vi "SampleCalibrationImages.vi"(7 "TLCamera reference in":refnum<k24>, 8 "Error In":errorcluster, 10 "ExposureTime_us":u32, 11 "MotorController in":refnum<class "MotorController.lvclass">) -> (0 "Error Out":errorcluster, 3 "MotorController out":refnum<class "MotorController.lvclass">, 5 "TLCamera reference out":refnum<k24>)   [LabVIEW 2019]
uses:
  SampleCalibrationCalculationResults_cluster_typedef.ctl
  MotorController.lvclass
  C:/Users/jleeman/git_repos/CAxis_Machine/C-Axis LabView Controller/Library_X64/Thorlabs.TSI.TLCameraInterfaces.dll
  Library_X64/Thorlabs.TSI.TLCameraInterfaces.dll
  SampleCalibration_enum_states_typedef.ctl
  Axes_enum_typedef.ctl
panel:
  out "Calculation Results":T1
  in  "Calculate":bool
  in  "Go":bool
  in  "Jog Sample Steps":i16
  in  "Image":bool
  in  "Next":bool
  out "Image 2":T2(plugin-control)
  out "Image 1":T2(plugin-control)
  # "Sample Calibration"
  # "Take photos of the grid at 0 and 180 degree stage positions, then compare the offsets of the grid dots. Jog the stage and repeat as desired until sample holder is level with respect to the camera."
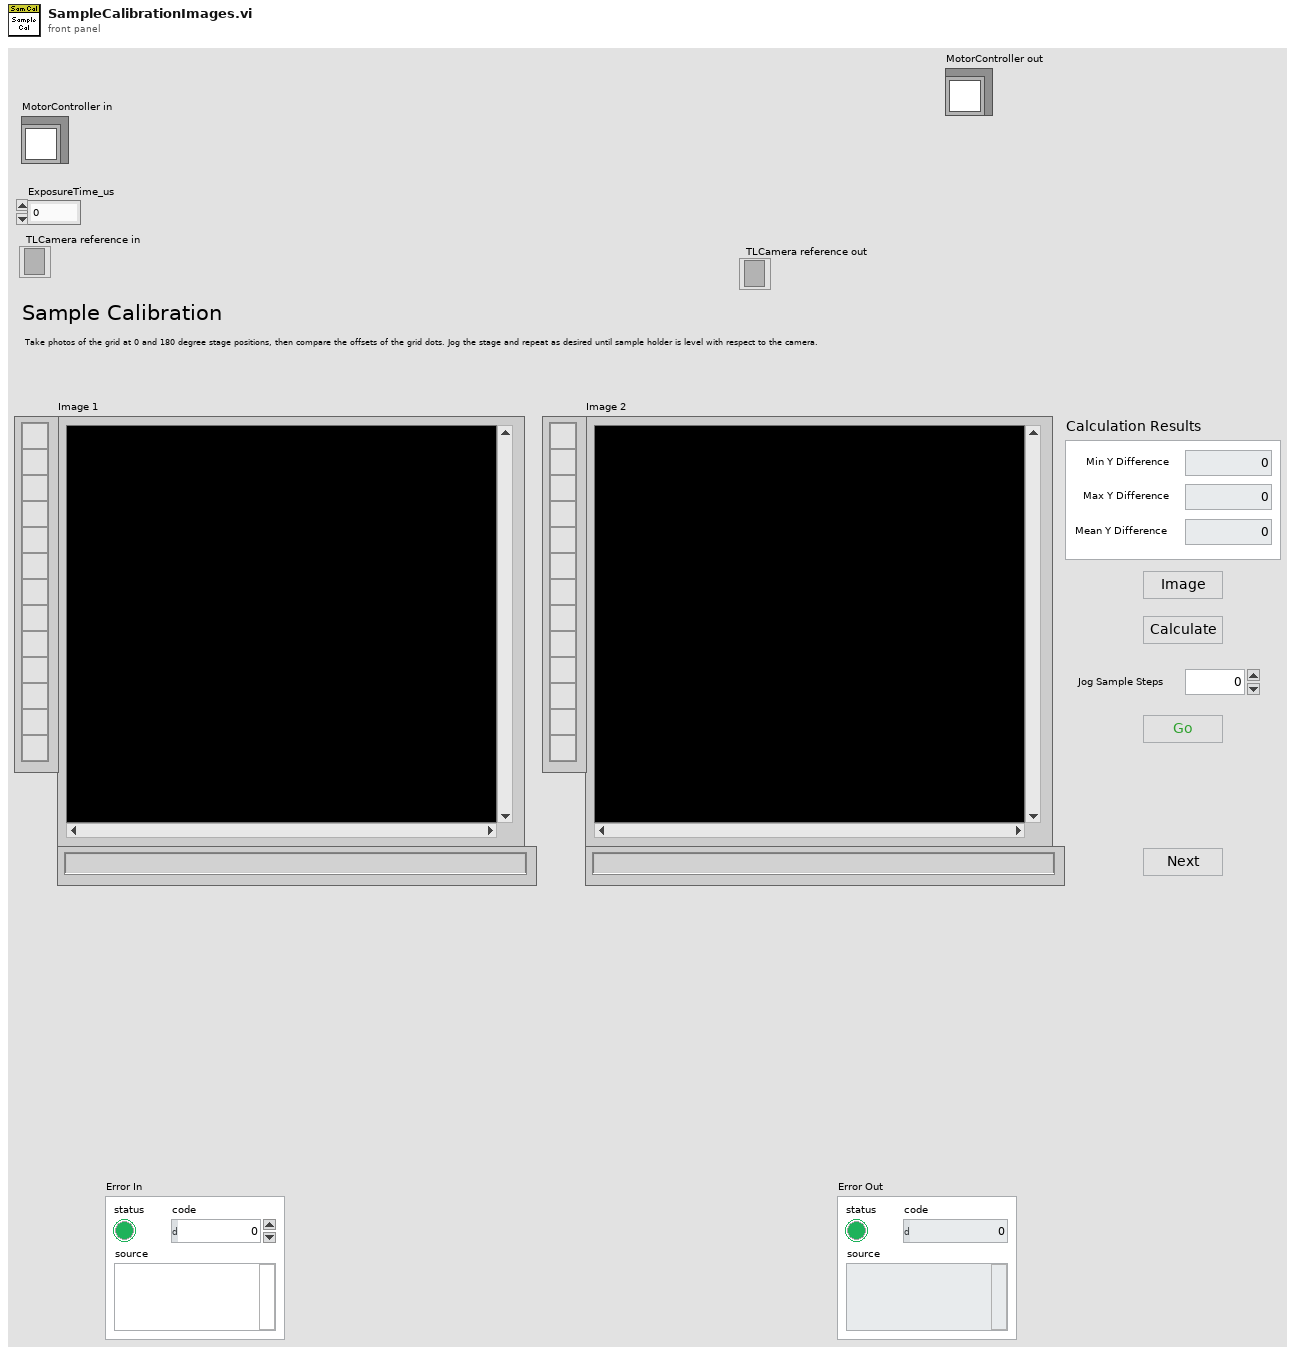
[diagram p1: front panel]
types:
  T1 = typedef "SampleCalibrationCalculationResults_cluster_typedef.ctl" = cluster{"Mean Y Difference":dbl, "Max Y Difference":dbl, "Min Y Difference":dbl}
  T2 = typedef "IMAQ Image.ctl" = refnum<image>
  T3 = typedef "Image Type" = u32
  T4 = enum8{"Enabled", "Disabled", "Disabled and Grayed Out"}
  T5 = typedef "SampleCalibration_enum_states_typedef.ctl" = enum16{"Initialize", "Move", "Capture", "Calculate", "Wait", "Shutdown"}
  T6 = typedef "Axes_enum_typedef.ctl" = enum16{"Polarizer 1", "Polarizer 2", "Sample", "Stage"}
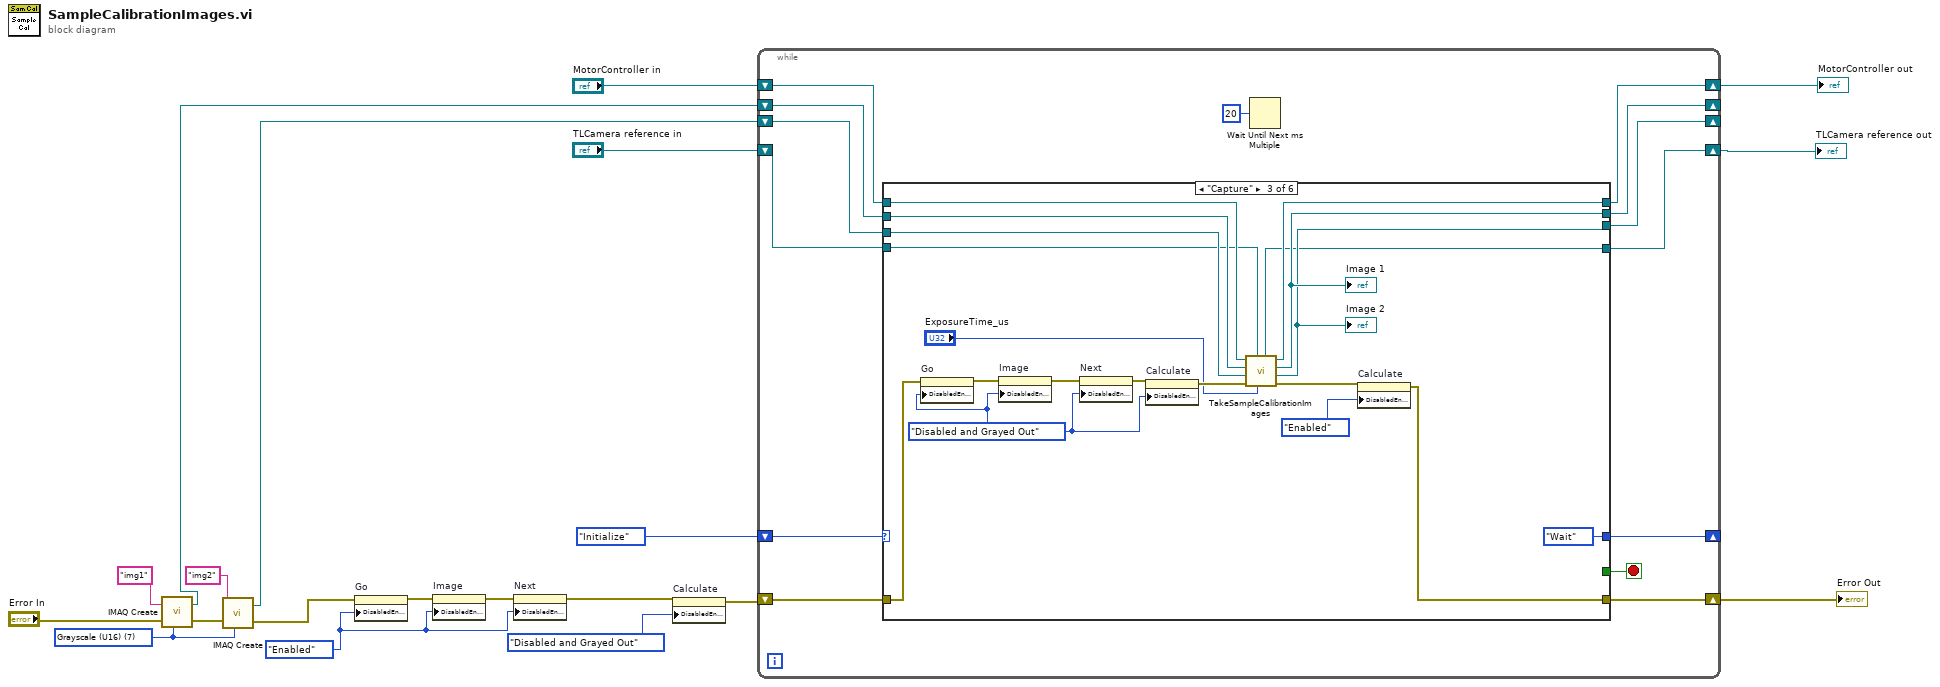
[diagram p0: block diagram]
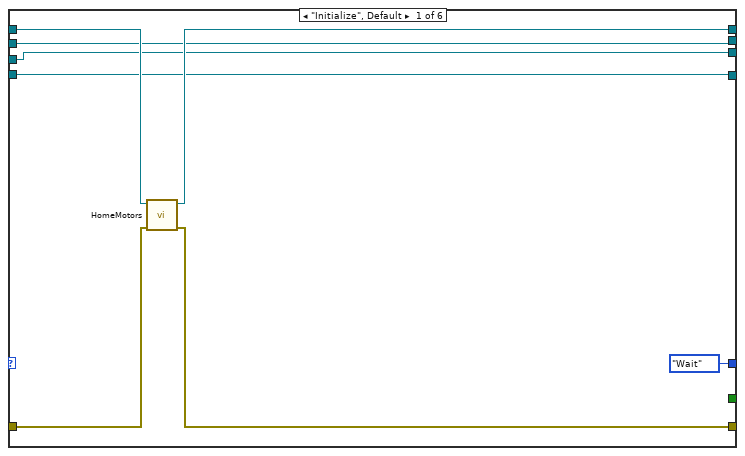
[diagram p2: hidden frame]
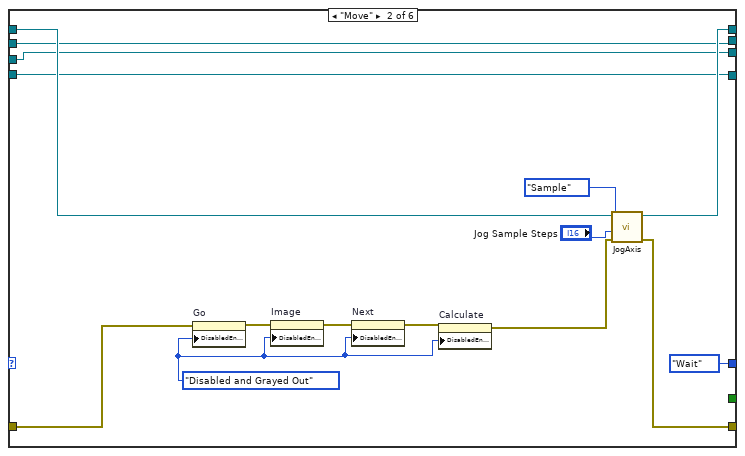
[diagram p3: hidden frame]
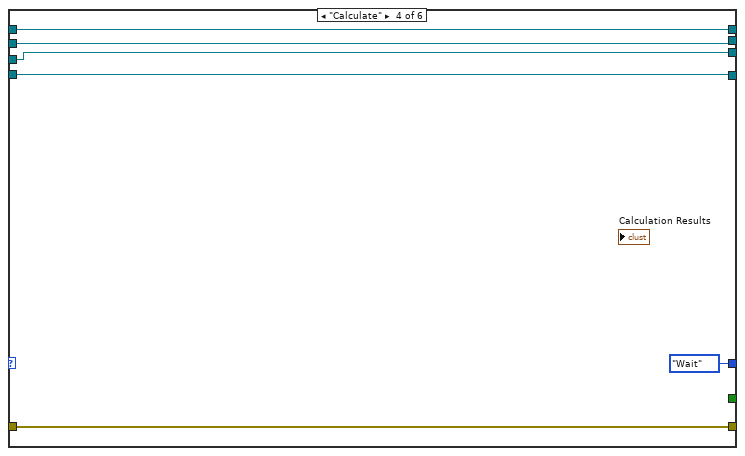
[diagram p4: hidden frame]
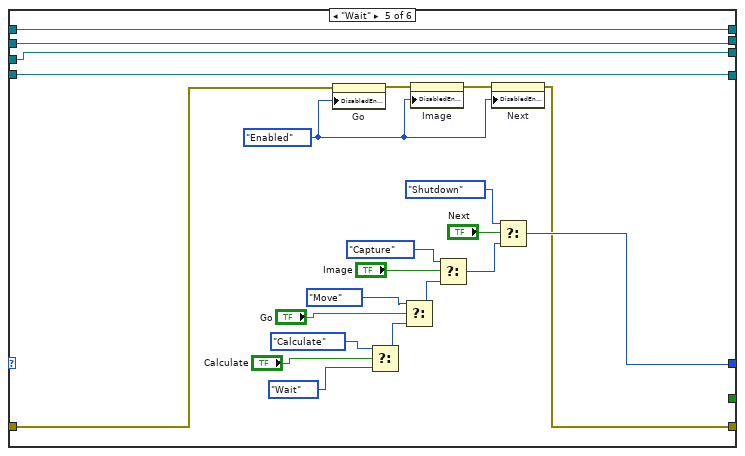
[diagram p5: hidden frame]
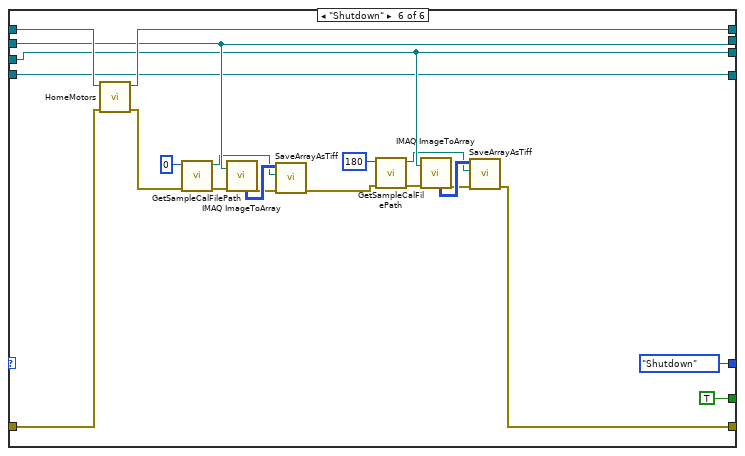
[diagram p6: hidden frame]
diagram:
  w1 = T3 7 items=["Grayscale (U8)", "Grayscale (I16)", "Grayscale (SGL)", "Complex (CSG)", "RGB (U32)", "HSL (U32)", "RGB (U64)", "Grayscale (U16)"] ("Image Type")
  w8 = T4."Enabled" ("Disabled")
  n1 = call "IMAQ Create"("Image Name"="img1", "Image Type"=w1, "error in (no error)"="Error In") -> ("New Image"=w12:T2, "error out"=w13:errorcluster)  [unwired: 2 in]
  n2 = call "IMAQ Create"("Image Name"="img2", "Image Type"=w1, "error in (no error)"=w13) -> ("New Image"=w11:T2, "error out"=w4:errorcluster)  [unwired: 2 in]
  n3 = property on="Go" class="Bool"(error in=w4, "DisabledEnum"=w8) -> (error out=w9:errorcluster)  [unwired: 1 in, 1 out]
  n4 = property on="Image" class="Bool"(error in=w9, "DisabledEnum"=w8) -> (error out=w10:errorcluster)  [unwired: 1 in, 1 out]
  n5 = property on="Next" class="Bool"(error in=w10, "DisabledEnum"=w8) -> (error out=w6:errorcluster)  [unwired: 1 in, 1 out]
  n6 = property on="Calculate" class="Bool"(error in=w6, "DisabledEnum"=T4."Disabled and Grayed Out" ("Disabled")) -> (error out=w5:errorcluster)  [unwired: 1 in, 1 out]
  n7 = while {
    shift-right: [w33] -> _
    shift-left: SampleCalibration_enum_states_typedef."Initialize" -> [w34]
    shift-right: [w31] -> w19
    shift-left: w5 -> [w32]
    shift-right: [w29] -> w17
    shift-left: "MotorController in" -> [w30]
    shift-right: [w26] -> _
    shift-left: w12 -> [w28]
    shift-right: [w25] -> _
    shift-left: w11 -> [w27]
    shift-right: [w21] -> w2
    shift-left: "TLCamera reference in" -> [w22]
    stop <- w24 stop-if-true
    n8 = case shown="\"Capture\"" w34 {
      tunnel: [SampleCalibration_enum_states_typedef."Wait" SampleCalibration_enum_states_typedef."Wait" SampleCalibration_enum_states_typedef."Wait" SampleCalibration_enum_states_typedef."Wait" w92 SampleCalibration_enum_states_typedef."Shutdown"] -> w33
      tunnel: w32 -> [w41 w47 w61 w81 w88 w123]
      tunnel: [w39 w53 w62 w81 w87 w106] -> w31
      tunnel: w30 -> [w42 w57 w70 w80 w86 w124]
      tunnel: [w40 w56 w69 w80 w86 w122] -> w29
      tunnel: w28 -> [w37 w45 w68 w79 w85 w120]
      tunnel: w27 -> [w36 w44 w67 w78 w84 w117]
      tunnel: [w37 w45 w65 w79 w85 w120] -> w26
      tunnel: [w36 w44 w64 w78 w84 w117] -> w25
      tunnel: [_ _ _ _ _ TRUE] -> w24
      tunnel: w22 -> [w35 w43 w59 w77 w83 w105]
      tunnel: [w35 w43 w58 w77 w83 w105] -> w21
      frame "Initialize", Default {
        n9 = call "HomeMotors.vi"("error in (no error)"=w41, "MotorController in"=w42) -> ("error out"=w39:errorcluster, "MotorController out"=w40:refnum<class "MotorController.lvclass">)  [unwired: 8 in]
      }
      frame "Move" {
        w48 = T4."Disabled and Grayed Out" ("Disabled")
        n10 = property on="Go" class="Bool"(error in=w47, "DisabledEnum"=w48) -> (error out=w50:errorcluster)  [unwired: 1 in, 1 out]
        n11 = property on="Image" class="Bool"(error in=w50, "DisabledEnum"=w48) -> (error out=w49:errorcluster)  [unwired: 1 in, 1 out]
        n12 = property on="Next" class="Bool"(error in=w49, "DisabledEnum"=w48) -> (error out=w51:errorcluster)  [unwired: 1 in, 1 out]
        n13 = property on="Calculate" class="Bool"(error in=w51, "DisabledEnum"=w48) -> (error out=w46:errorcluster)  [unwired: 1 in, 1 out]
        n14 = call "JogAxis.vi"("error in (no error)"=w46, "Steps"="Jog Sample Steps", "Axis"=Axes_enum_typedef."Sample", "MotorController in"=w57) -> ("error out"=w53:errorcluster, "MotorController out"=w56:refnum<class "MotorController.lvclass">)  [unwired: 6 in]
      }
      frame "Capture" {
        w71 = T4."Disabled and Grayed Out" ("Disabled")
        n15 = property on="Go" class="Bool"(error in=w61, "DisabledEnum"=w71) -> (error out=w73:errorcluster)  [unwired: 1 in, 1 out]
        n16 = property on="Image" class="Bool"(error in=w73, "DisabledEnum"=w71) -> (error out=w74:errorcluster)  [unwired: 1 in, 1 out]
        n17 = property on="Next" class="Bool"(error in=w74, "DisabledEnum"=w71) -> (error out=w72:errorcluster)  [unwired: 1 in, 1 out]
        n18 = property on="Calculate" class="Bool"(error in=w72, "DisabledEnum"=w71) -> (error out=w66:errorcluster)  [unwired: 1 in, 1 out]
        n19 = call "TakeSampleCalibrationImages.vi"("ExposureTime_us"="ExposureTime_us", "TLCamera reference in"=w59, "Error In"=w66, "Img2 in"=w67, "Img1 in"=w68, "MotorController in"=w70) -> ("Error Out"=w63:errorcluster, "Img2 out"=w64:T2, "Img1 out"=w65:T2, "MotorController out"=w69:refnum<class "MotorController.lvclass">, "TLCamera reference out"=w58:refnum<k24>)  [unwired: 1 in]
        "Image 1" <- w65
        "Image 2" <- w64
        n20 = property on="Calculate" class="Bool"(error in=w63, "DisabledEnum"=T4."Enabled" ("Disabled")) -> (error out=w62:errorcluster)  [unwired: 1 in, 1 out]
      }
      frame "Calculate" {
      }
      frame "Wait" {
        w89 = T4."Enabled" ("Disabled")
        n21 = property on="Go" class="Bool"(error in=w88, "DisabledEnum"=w89) -> (error out=w90:errorcluster)  [unwired: 1 in, 1 out]
        n22 = Select(t=SampleCalibration_enum_states_typedef."Calculate", s="Calculate", f=SampleCalibration_enum_states_typedef."Wait") -> (s? t:f=w103:T5)
        n23 = Select(t=SampleCalibration_enum_states_typedef."Move", s="Go", f=w103) -> (s? t:f=w102:T5)
        n24 = property on="Image" class="Bool"(error in=w90, "DisabledEnum"=w89) -> (error out=w91:errorcluster)  [unwired: 1 in, 1 out]
        n25 = Select(t=SampleCalibration_enum_states_typedef."Capture", s="Image", f=w102) -> (s? t:f=w101:T5)
        n26 = property on="Next" class="Bool"(error in=w91, "DisabledEnum"=w89) -> (error out=w87:errorcluster)  [unwired: 1 in, 1 out]
        n27 = Select(t=SampleCalibration_enum_states_typedef."Shutdown", s="Next", f=w101) -> (s? t:f=w92:T5)
      }
      frame "Shutdown" {
        n28 = call "HomeMotors.vi"("error in (no error)"=w123, "MotorController in"=w124) -> ("error out"=w107:errorcluster, "MotorController out"=w122:refnum<class "MotorController.lvclass">)  [unwired: 8 in]
        n29 = call "GetSampleCalFilePath.vi"("Error In"=w107, "Position"=i16 0) -> ("Error Out"=w114:errorcluster, "path"=w112:path)  [unwired: 8 in]
        n30 = call "IMAQ ImageToArray"("error in (no error)"=w114, "Image"=w120) -> ("Image Pixels (U16)"=w119:u16[][], "error out"=w118:errorcluster)  [unwired: 2 in, 3 out]
        n31 = call "SaveArrayAsTiff.vi"("Error In"=w118, "File Path"=w112, "Array"=w119) -> ("Error Out"=w108:errorcluster)  [unwired: 7 in, 1 out]
        n32 = call "GetSampleCalFilePath.vi"("Error In"=w108, "Position"=i16 180) -> ("Error Out"=w110:errorcluster, "path"=w109:path)  [unwired: 8 in]
        n33 = call "IMAQ ImageToArray"("error in (no error)"=w110, "Image"=w117) -> ("Image Pixels (U16)"=w116:u16[][], "error out"=w115:errorcluster)  [unwired: 2 in, 3 out]
        n34 = call "SaveArrayAsTiff.vi"("Error In"=w115, "File Path"=w109, "Array"=w116) -> ("Error Out"=w106:errorcluster)  [unwired: 7 in, 1 out]
      }
    }
    n35 = Wait Until Next ms Multiple(millisecond multiple=u32 20) -> ()  [unwired: 1 out]
  }
  "Error Out" <- w19
  "MotorController out" <- w17
  "TLCamera reference out" <- w2
